vi "Get Current Match from XML.vi"(11 "XML In":string) -> (3 "Current Match":string)   [LabVIEW 2013]
uses:
  <vilib>/xml/Close Reference(Node).vi
  <vilib>/xml/NI_XML.lvlib
  <resource>/objmgr/DOMUserDefRef.rc
panel:
  out "error out":errorcluster
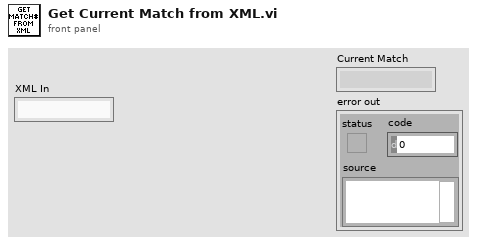
[diagram p1: front panel]
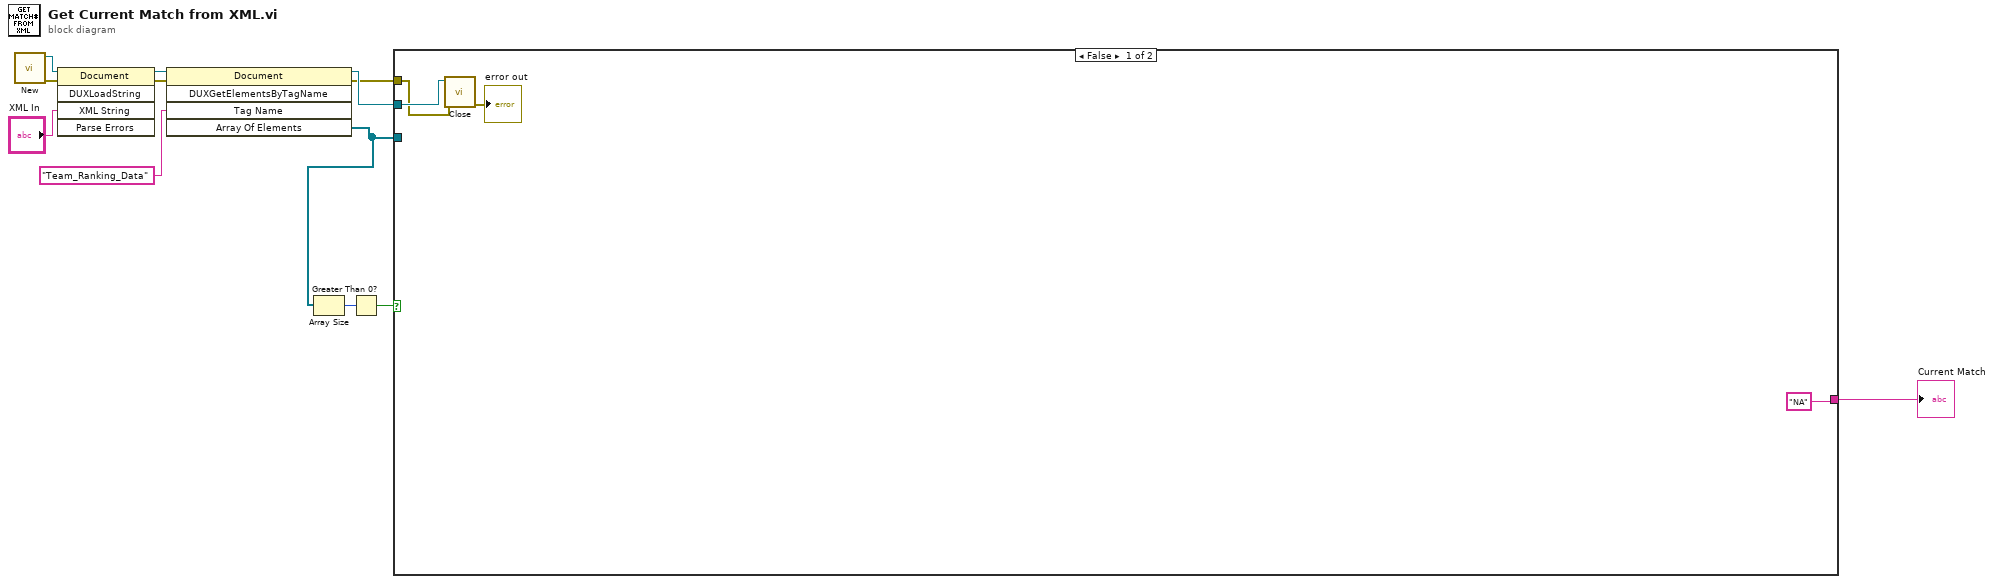
[diagram p0: block diagram]
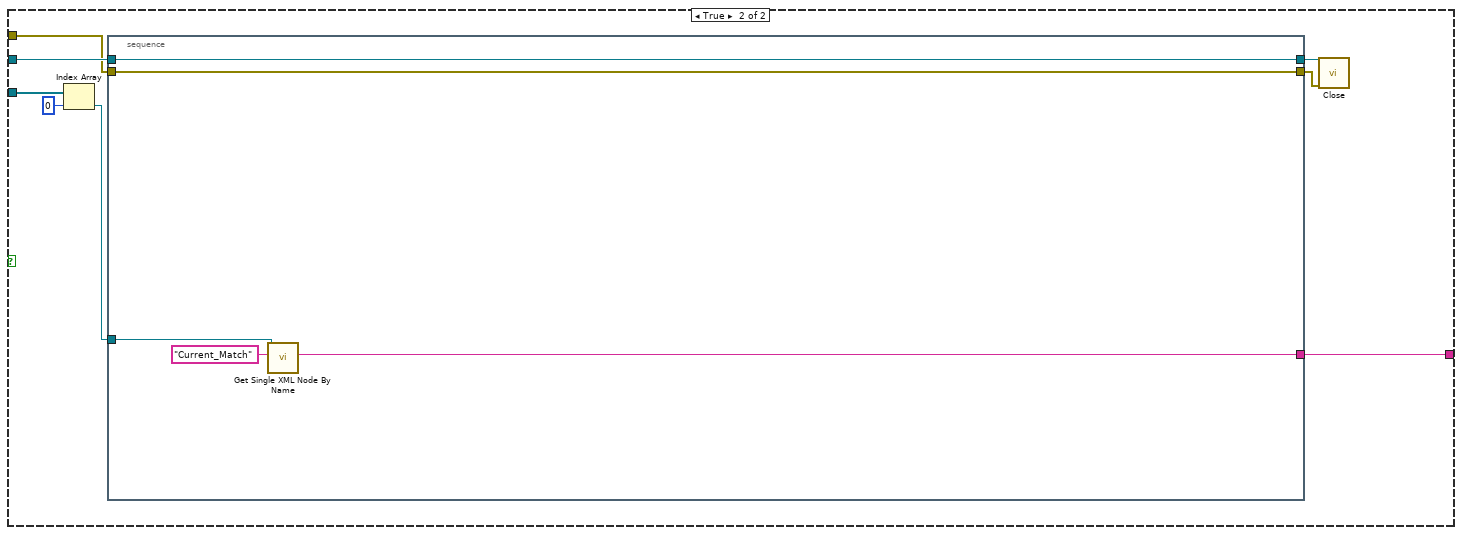
[diagram p2: hidden frame]
diagram:
  n1 = call <vilib>:"New.vi"() -> ("error out"=w7:errorcluster, "DOM document out"=w10:refnum<k20>)  [unwired: 8 in]
  n2 = invoke class="Document" method="DUXLoadString"(reference=w10, error in=w7, "XML String"="XML In") -> (reference out=w9:refnum<k20>, error out=w8:errorcluster)  [unwired: 2 in, 3 out]
  n3 = invoke class="Document" method="DUXGetElementsByTagName"(reference=w9, error in=w8, "Tag Name"="Team_Ranking_Data") -> (reference out=w6:refnum<k20>, error out=w5:errorcluster, "Array Of Elements"=w1:refnum<k20>[])  [unwired: 2 in, 2 out]
  n4 = Array Size(array=w1) -> (size(s)=w2:i32)
  n5 = Greater Than 0?(x=w2) -> (x > 0?=w3:bool)
  n6 = case shown="False" w3 {
    tunnel: w6 -> [w16 w22]
    tunnel: w5 -> [w15 w21]
    tunnel: w1 -> [_ w20]
    tunnel: ["NA" w17] -> w4
    frame False {
      n7 = call-poly <vilib>:"Close.vi"("error in (no error)"=w15, "node"=w16) -> ("error out"=→"error out":errorcluster)  [unwired: 7 in]
    }
    frame True {
      n8 = Index Array(array=w20, index=0) -> (element=w18:refnum<k20>)
      n9 = stacked-sequence {
        tunnel: w18 -> [w27]
        tunnel: w22 -> [w29]
        tunnel: [w29] -> w24
        tunnel: w21 -> [w28]
        tunnel: [w28] -> w23
        tunnel: [w25] -> w17
        frame #0 {
          n10 = call "Get Single XML Node By Name.vi"("Tag Name"="Current_Match", "Parent Element"=w27) -> ("node text"=w25:string)  [unwired: 7 in, 2 out]
        }
      }
      n11 = call-poly <vilib>:"Close.vi"("error in (no error)"=w23, "node"=w24) -> ()  [unwired: 7 in, 1 out]
    }
  }
  "Current Match" <- w4
